vi "Debug Info Display.vi"(0 "Tamer in":refnum<class "Tamer.lvclass">, 11 "error in (no error)":errorcluster, 12 "Do not clear":bool=TRUE) -> (4 "Tamer out":refnum<class "Tamer.lvclass">, 15 "error out":errorcluster)   [LabVIEW 2020, in "TALOS.lvlib" / "Tamer.lvlib" / "Tamer.lvclass"]
uses:
  Tamer.lvclass
  Run Utilities/TypeDefs/Synchronize FPGA Cluster.ctl
  Run Utilities/TypeDefs/Messages/Banana Message.ctl
  Run Utilities/TypeDefs/Return Code.ctl
  Run Utilities/TypeDefs/Monkey Status.ctl
  Highlighted string.ctl
  Run Utilities/TypeDefs/Messages/Script Checker Message.ctl
  Run Utilities/TypeDefs/Script Checker Result.ctl
  Tamer.lvclass/Tamer.ctl
  2837e8c5-8372-48ed-a217-086841ba2b74.vi
  095c6f48-196e-464b-ab3d-ae951524fe50.vi
  4905ac96-b208-4a41-83cc-f8013deddd10.vi
  58ee45cc-7794-4f39-a2fa-ddaa144d4c77.vi
  <vilib>/Comparison/Less/Less Functor/Less Functor.lvclass
  Run Utilities/Run Utilities.lvlib
panel:
  out "Global Status":bool
  out "Stopped":bool
  in  "Tab Control":T1(tab)
  out "Processes":map{string, string[]}(c390)
  out "Monkeys Status":map{string, T2}(c390)
  out "Monkeys":map{string, string[]}(c390)
  out "Kaslis":map{string, string}(c390)
  out "Checker Messages":T3[](array[typedef])
  out "Bananas":T5[](array[typedef])
  out "Sync. Mask":T7[](array[typedef])
  out "uServices replies":T8[](array[typedef])
  out "Guardians replies":T8[](array[typedef])
  # "No-Go"
  # "Go"
  # "No response"
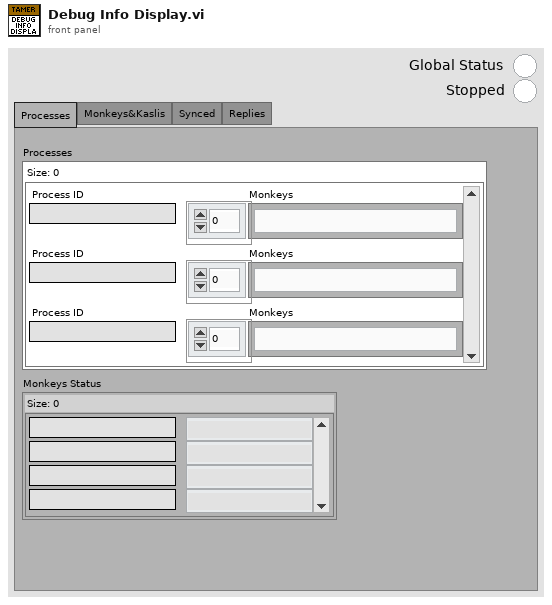
[diagram p1: front panel]
types:
  T1 = enum32{"Processes", "Monkeys&Kaslis", "Synced", "Replies"}
  T2 = typedef "TALOS.lvlib/Run Utilities.lvlib/Monkey Status.ctl" = enum16{"Init", "Paused", "Ongoing", "Stopped", "Finished (no errors)", "Finished (with errors)"}
  T3 = typedef "TALOS.lvlib/Run Utilities.lvlib/Script Checker Message.ctl" = cluster{"Monkey ID":string, "Script Checker Result":T4}
  T4 = typedef "TALOS.lvlib/Run Utilities.lvlib/Script Checker Result.ctl" = enum16{"Passed", "Failed", "Empty"}
  T5 = typedef "TALOS.lvlib/Run Utilities.lvlib/Banana Message.ctl" = cluster{"FPGA Name":string, "Return Code":T6}
  T6 = typedef "TALOS.lvlib/Run Utilities.lvlib/Return Code.ctl" = enum16{"All Good", "Retry", "Skip", "Skip All", "ABORT"}
  T7 = typedef "TALOS.lvlib/Run Utilities.lvlib/Synchronize FPGA Cluster.ctl" = cluster{"Status":bool, "FPGA Name":string}
  T8 = typedef "TALOS.lvlib/Tamer.lvlib/Tamer.lvclass/Highlighted string.ctl" = cluster{"Highlight":u32, "String":string}
  T9 = typedef "TALOS.lvlib/Tamer.lvlib/Tamer.lvclass/Reply.ctl" = cluster{"ID":string, "Status":bool, "GUID":string}
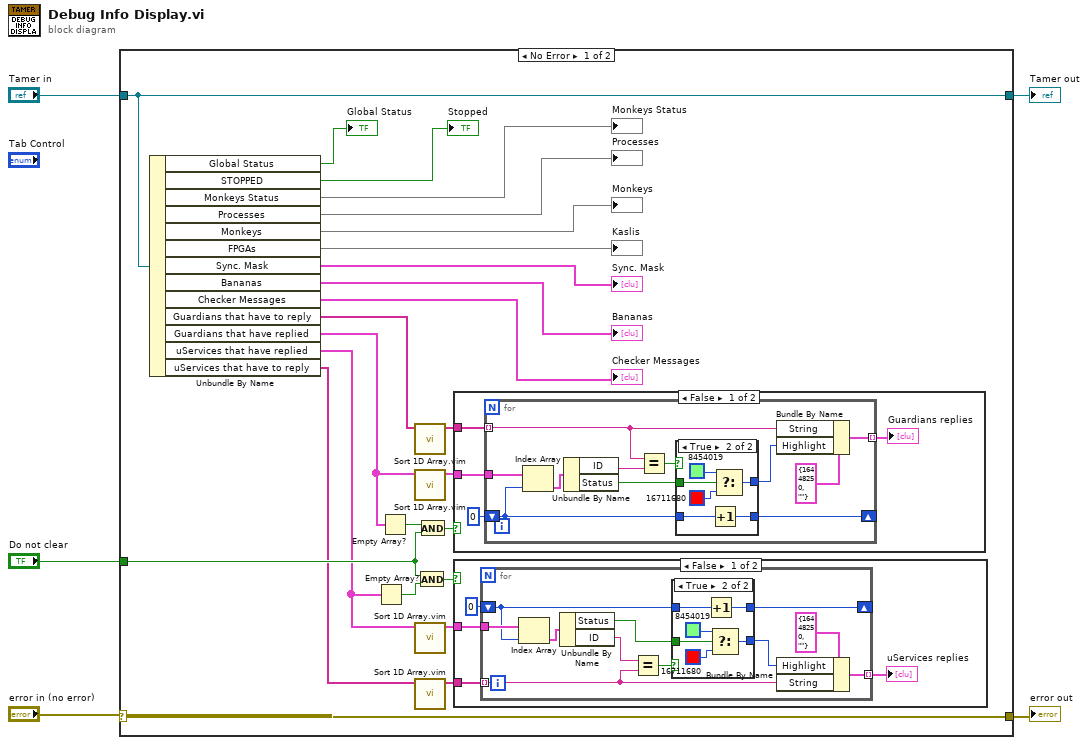
[diagram p0: block diagram]
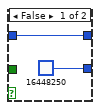
[diagram p2: hidden frame]
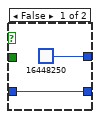
[diagram p4: hidden frame]
diagram:
  n1 = case shown="No Error" "error in (no error)" {
    selector: "error in (no error)" -> [w18 w76]
    tunnel: "Tamer in" -> [w19 w77]
    tunnel: [w19 w77] -> w5
    tunnel: [w18 w76] -> w3
    tunnel: "Do not clear" -> [w21 _]
    frame No Error {
      n2 = Unbundle By Name(w19) -> ("Global Status"=→"Global Status":bool, "STOPPED"=→"Stopped":bool, "Monkeys Status"=→"Monkeys Status":map{string, T2}, "Processes"=→"Processes":map{string, string[]}, "Monkeys"=→"Monkeys":map{string, string[]}, "FPGAs"=→"Kaslis":map{string, string}, "Sync. Mask"=→"Sync. Mask":T7[], "Bananas"=→"Bananas":T5[], "Checker Messages"=→"Checker Messages":T3[], "Guardians that have to reply"=w13:string[], "Guardians that have replied"=w15:T9[], "uServices that have replied"=w10:T9[], "uServices that have to reply"=w8:string[])
      n3 = Empty Array?(array=w10) -> (empty?=w22:bool)
      n4 = Empty Array?(array=w15) -> (empty?=w24:bool)
      n5 = call "Sort 1D Array.vim"("unsorted array"=w13) -> ("sorted array"=w12:string[])  [unwired: 10 in]
      n6 = call "Sort 1D Array.vim"("unsorted array"=w15) -> ("sorted array"=w14:T9[])  [unwired: 10 in]
      n7 = call "Sort 1D Array.vim"("unsorted array"=w10) -> ("sorted array"=w9:T9[])  [unwired: 10 in]
      n8 = call "Sort 1D Array.vim"("unsorted array"=w8) -> ("sorted array"=w7:string[])  [unwired: 10 in]
      n9 = And(x=w21, y=w22) -> (x .and. y?=w11:bool)
      n10 = And(x=w24, y=w21) -> (x .and. y?=w25:bool)
      n11 = case shown="False" w25 {
        tunnel: w14 -> [w55 _]
        tunnel: w12 -> [w56 _]
        frame False {
          n12 = for {
            tunnel: w56 -> [w59] mode=indexing
            tunnel: w55 -> [w64]
            shift-right: [w62] -> _
            shift-left: 0 -> [w61]
            tunnel: [w57] -> w53 mode=indexing
            n13 = Index Array(array=w64, index=w61) -> (element=w63:T9)
            n14 = Unbundle By Name(w63) -> ("ID"=w67:string, "Status"=w65:bool)
            n15 = Equal?(x=w59, y=w67) -> (x = y?=w66:bool)
            n16 = case shown="True" w66 {
              tunnel: w65 -> [_ w72]
              tunnel: [w69 w75] -> w62
              tunnel: w61 -> [w69 w74]
              tunnel: [u32 16448250 ("Highlight") w73] -> w58
              frame False {
              }
              frame True {
                n17 = Increment(x=w74) -> (x+1=w75:i32)
                n18 = Select(t=u32 8454019 ("Highlight"), s=w72, f=u32 16711680 ("Color")) -> (s? t:f=w73:u32)
              }
            }
            n19 = Bundle By Name(cluster=T8 {"Highlight"=16448250, "String"=""} ("Highlited string"), "String"=w59, "Highlight"=w58) -> (w57:T8)
          }
          "Guardians replies" <- w53
        }
        frame True {
        }
      }
      n20 = case shown="False" w11 {
        tunnel: w9 -> [w33 _]
        tunnel: w7 -> [w30 _]
        frame False {
          n21 = for {
            tunnel: w30 -> [w34] mode=indexing
            tunnel: w33 -> [w43]
            shift-right: [w41] -> _
            shift-left: 0 -> [w40]
            tunnel: [w38] -> w31 mode=indexing
            n22 = Index Array(array=w43, index=w40) -> (element=w42:T9)
            n23 = Unbundle By Name(w42) -> ("Status"=w36:bool, "ID"=w37:string)
            n24 = Equal?(x=w37, y=w34) -> (x = y?=w44:bool)
            n25 = case shown="True" w44 {
              tunnel: w36 -> [_ w49]
              tunnel: [w46 w52] -> w41
              tunnel: w40 -> [w46 w51]
              tunnel: [u32 16448250 ("Highlight") w50] -> w35
              frame False {
              }
              frame True {
                n26 = Increment(x=w51) -> (x+1=w52:i32)
                n27 = Select(t=u32 8454019 ("Highlight"), s=w49, f=u32 16711680 ("Color")) -> (s? t:f=w50:u32)
              }
            }
            n28 = Bundle By Name(cluster=T8 {"Highlight"=16448250, "String"=""} ("Highlited string"), "Highlight"=w35, "String"=w34) -> (w38:T8)
          }
          "uServices replies" <- w31
        }
        frame True {
        }
      }
    }
    frame Error {
    }
  }
  "error out" <- w3
  "Tamer out" <- w5
